vi "Range_to_memory_address_CH1.vi"(11 "INPUT2 CH1 Range IN":dbl) -> (0 "LB address":string, 1 "HB address":string, 2 "UB address":string, 3 "MB address":string, 4 "Sign Addrss":string)   [LabVIEW 2012]
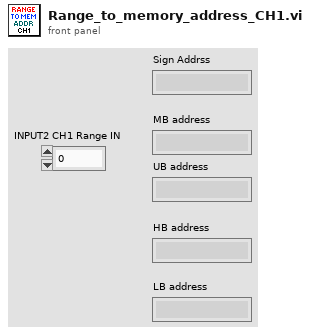
[diagram p1: front panel]
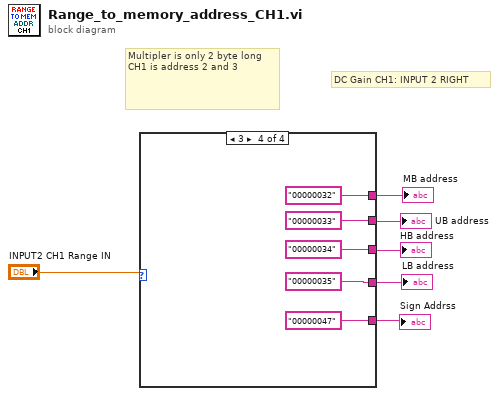
[diagram p0: block diagram]
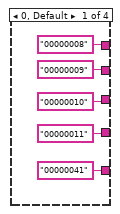
[diagram p2: hidden frame]
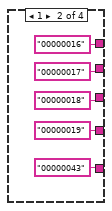
[diagram p3: hidden frame]
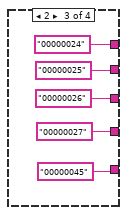
[diagram p4: hidden frame]
diagram:
  # "DC Gain CH1: INPUT 2 RIGHT"
  # "Multipler is only 2 byte long \nCH1 is address 2 and 3"
  n1 = case shown="3" "INPUT2 CH1 Range IN" {
    tunnel: ["00000008" "00000016" "00000024" "00000032"] -> w5
    tunnel: ["00000009" "00000017" "00000025" "00000033"] -> w4
    tunnel: ["00000010" "00000018" "00000026" "00000034"] -> w3
    tunnel: ["00000011" "00000019" "00000027" "00000035"] -> w2
    tunnel: ["00000041" "00000043" "00000045" "00000047"] -> w1
    frame 0, Default {
    }
    frame 1 {
    }
    frame 2 {
    }
    frame 3 {
    }
  }
  "MB address" <- w5
  "UB address" <- w4
  "HB address" <- w3
  "LB address" <- w2
  "Sign Addrss" <- w1
